vi "CRYDataView Pic LIB.vi"(7 "sAction":string, 8 "nData":i32, 9 "sData":string, 10 "sOption":string, 11 "cView":T1) -> (0 "nData_Out":i32, 1 "sData_Out":string, 3 "cView_Out":T1)   [LabVIEW 2013]
uses:
  Control/CRYGraph Property.ctl
  SubVI/CRYMain Sub Window Global.vi
  CRYMainGlobal.vi
  CRYProject/CRYProject Editor Global.vi
panel:
  in  "bWait":bool=TRUE
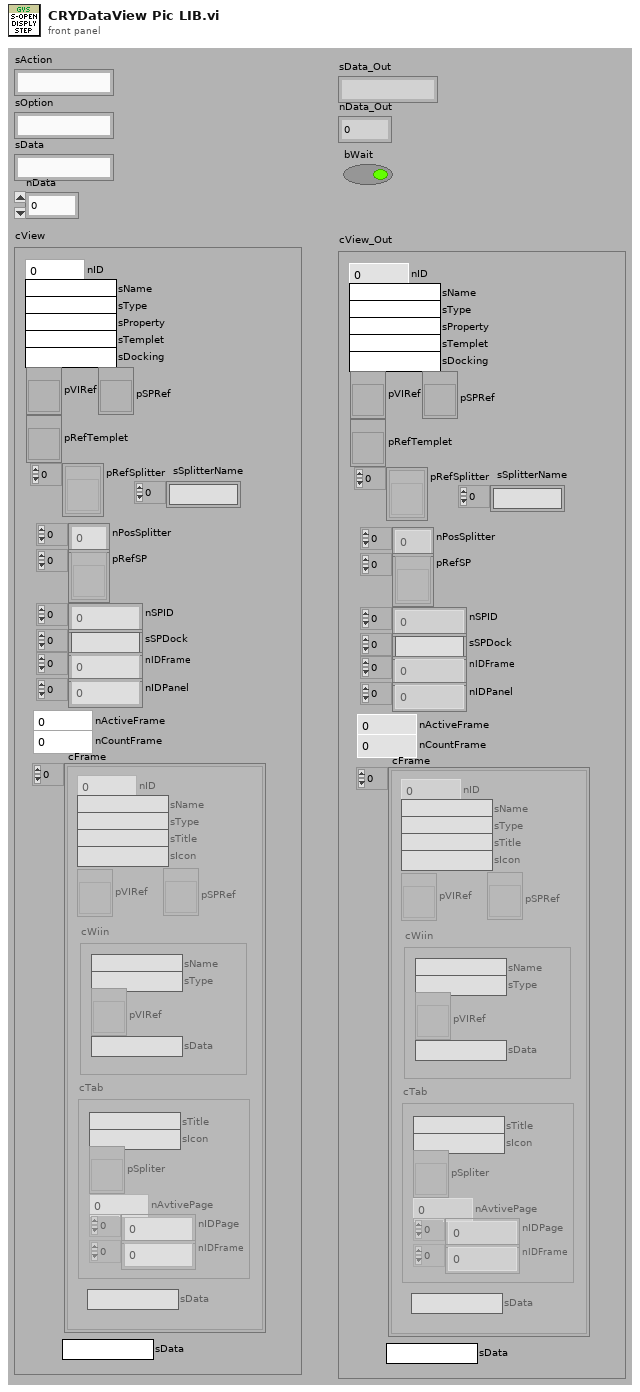
[diagram p1: front panel]
types:
  T1 = cluster{"nID":i32, "sName":string, "sType":string, "sProperty":string, "sTemplet":string, "sDocking":string, "pVIRef":refnum<vi>, "pSPRef":refnum<vi>, "pRefTemplet":refnum<vi>, "pRefSplitter":refnum<vi>[], "nPosSplitter":i32[], "pRefSP":refnum<vi>[], "nSPID":i32[], "sSPDock":string[], "nIDFrame":i32[], "nIDPanel":i32[], "nActiveFrame":i32, "nCountFrame":i32, "cFrame":cluster{"nID":i32, "sName":string, "sType":string, "sTitle":string, "sIcon":string, "pVIRef":refnum<vi>, "pSPRef":refnum<vi>, "cWiin":cluster{"sName":string, "sType":string, "pVIRef":refnum<vi>, "sData":string}, "cTab":cluster{"sTitle":string, "sIcon":string, "pSpliter":refnum<vi>, "nAvtivePage":i32, "nIDPage":i32[], "nIDFrame":i32[]}, "sData":string}[], "sData":string, "sSplitterName":string[]}
  T2 = typedef "CRYGraph Property.ctl" = cluster{"LegendShow":bool, "Legend Splitter Position":dbl, "Data Names":string[], "Item Symbols":i32[], "Color Array":u32[], "Flattened Plot Property":string, "CursorShow":bool, "Flattened Cursor Property":string, "Graph Number":i32, "Flattened Scale Property":string, "PreviewShow":bool, "MagnitudeShow":bool, "PaletteShow":bool, "XYShow":bool, "FrequencyShow":bool, "Frequency Splitter Position":dbl, "XYGraph Splitter Position":dbl, "Frequency Symbols":i32[], "LegendVScrollShow":bool, "FrequencyVScrollShow":bool, "PhaseShow":bool, "Title Name":string}
  T3 = typedef "LVRectTypeDef.ctl" = cluster{"Left":i16, "Top":i16, "Right":i16, "Bottom":i16}
  T4 = cluster{"nID":i32[], "Frame":cluster{"nType":i32, "nParent":i32, "pVIW":refnum<vi>, "pSPW":refnum<vi>, "nTypeF":i32, "pVIF":refnum<vi>, "pSPF":refnum<vi>, "nIDSpliter":i32, "nProperty":i32, "Bound":T3, "nID":i32, "nData":i32, "sData":string, "pWVI":refnum<vi>, "sTitle":string, "cPages":cluster{"nPage":i32, "sTitle":string, "sIcon":string, "pVI":refnum<vi>, "nID":i32}[], "pTab":refnum<vi>, "nIDPages":i32[], "pSPT":refnum<vi>, "sTemp":string, "nDockID":i32, "nDockLR":i32, "sIcon":string}[]}
  T5 = cluster{"nType":i32, "nParent":i32, "pVIW":refnum<vi>, "pSPW":refnum<vi>, "nTypeF":i32, "pVIF":refnum<vi>, "pSPF":refnum<vi>, "nIDSpliter":i32, "nProperty":i32, "Bound":T3, "nID":i32, "nData":i32, "sData":string, "pWVI":refnum<vi>, "sTitle":string, "cPages":cluster{"nPage":i32, "sTitle":string, "sIcon":string, "pVI":refnum<vi>, "nID":i32}[], "pTab":refnum<vi>, "nIDPages":i32[], "pSPT":refnum<vi>, "sTemp":string, "nDockID":i32, "nDockLR":i32, "sIcon":string}[]
  T6 = typedef "CRYTS.ctl" = cluster{"No.TS":u16, "TS File Path":path, "TS Name":string, "EditStepName":string, "Steps":T7[], "New State":bool, "Change State":bool, "Flattened CurveLib Data":string, "Document Data":string, "EditStepNo":u16, "Operator Start File":string, "Sequence Type":string, "Sequence Language":string}
  T7 = typedef "CRYStep.ctl" = cluster{"No.VI":i32, "Category":string, "StepName":string, "Seq setup flattened":string, "Comment":string, "Steps config.":bool[], "Jump config":i32[], "Start":dbl, "Increment":dbl, "Name":string, "Unit":string, "Y data":u16, "Y prefix":string, "Y dB ref":dbl, "Y unit":string, "Repeat State Array":cluster{"Start":dbl, "Increment":dbl, "Count":i32, "Num":i32}[]}
  T8 = cluster{"nType":i32, "nParent":i32, "pVIW":refnum<vi>, "pSPW":refnum<vi>, "nTypeF":i32, "pVIF":refnum<vi>, "pSPF":refnum<vi>, "nIDSpliter":i32, "nProperty":i32, "Bound":T3, "nID":i32, "nData":i32, "sData":string, "pWVI":refnum<vi>, "sTitle":string, "cPages":cluster{"nPage":i32, "sTitle":string, "sIcon":string, "pVI":refnum<vi>, "nID":i32}[], "pTab":refnum<vi>, "nIDPages":i32[], "pSPT":refnum<vi>, "sTemp":string, "nDockID":i32, "nDockLR":i32, "sIcon":string}
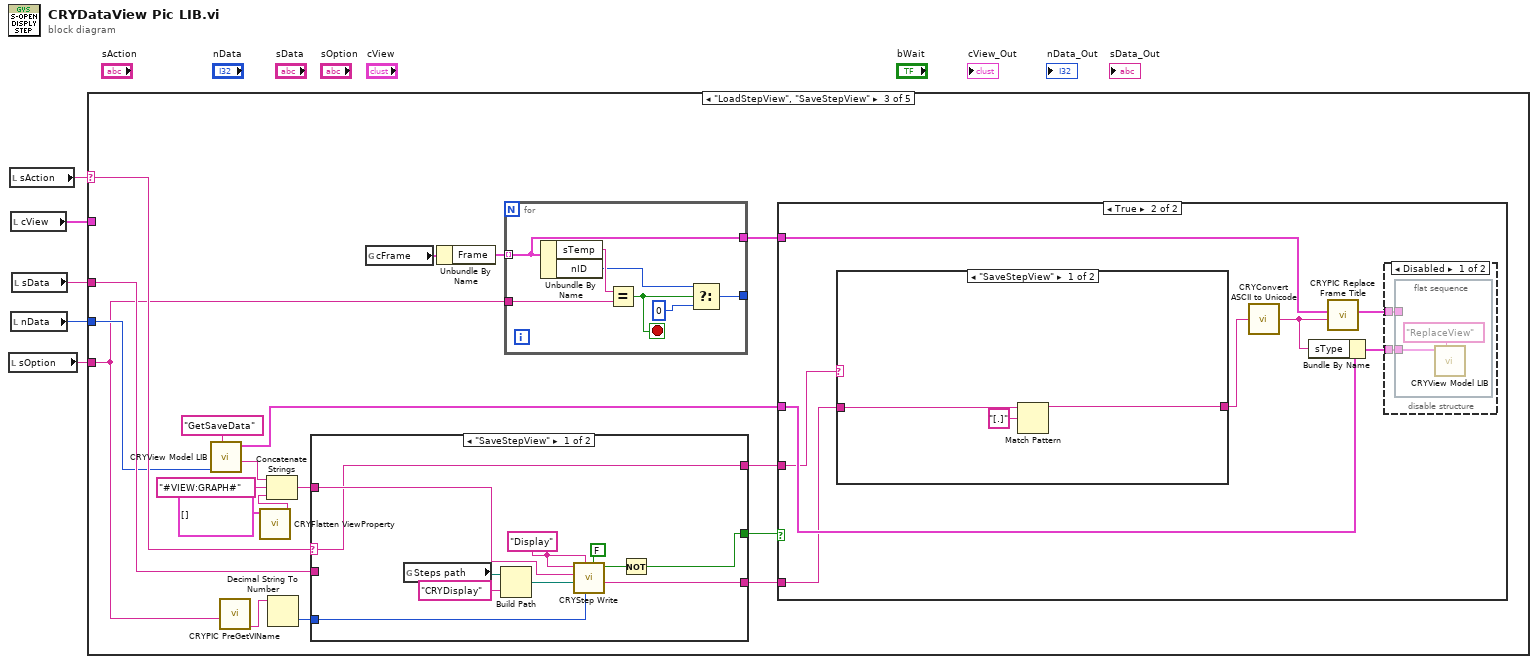
[diagram p0: block diagram]
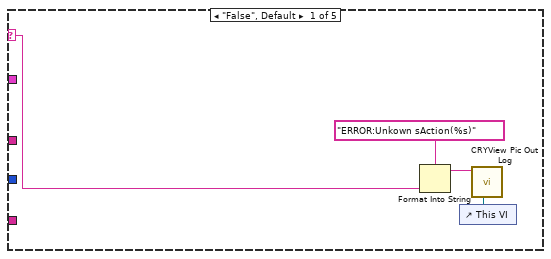
[diagram p2: hidden frame]
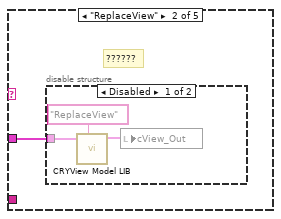
[diagram p3: hidden frame]
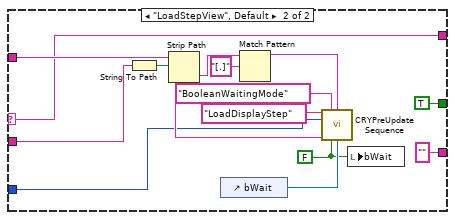
[diagram p5: hidden frame]
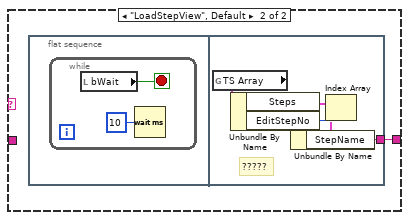
[diagram p8: hidden frame]
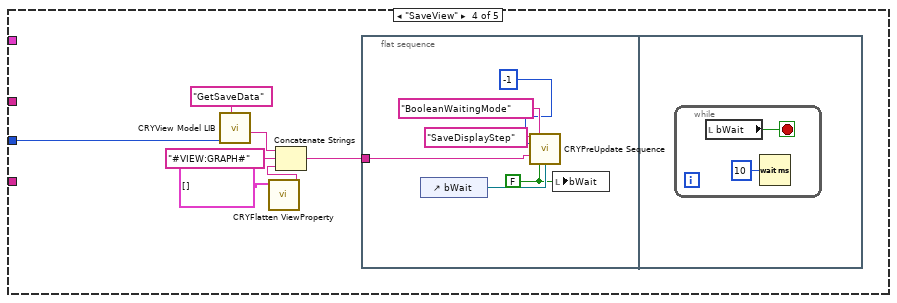
[diagram p9: hidden frame]
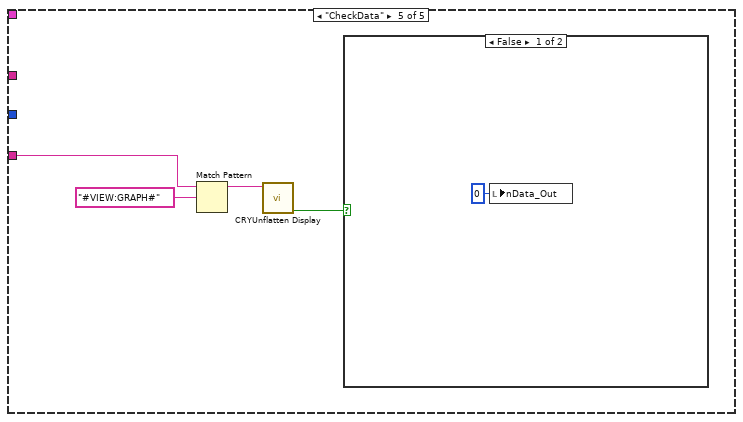
[diagram p10: hidden frame]
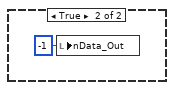
[diagram p11: hidden frame]
diagram:
  n1 = local read "sOption"() -> (w2:string)
  n2 = local read "sAction"() -> (w5:string)
  n3 = local read "cView"() -> (w1:T1)
  n4 = local read "nData"() -> (w3:i32)
  n5 = local read "sData"() -> (w4:string)
  n6 = case shown="\"LoadStepView\", \"SaveStepView\"" w5 {
    selector: w5 -> [w7 _ w28 _ _]
    tunnel: w4 -> [_ _ w29 _ _]
    tunnel: w3 -> [_ _ w22 w89 _]
    tunnel: w2 -> [_ _ w17 _ w105]
    tunnel: w1 -> [_ w10 _ _ _]
    frame "False", Default {
      n7 = Format Into String(format string="ERROR:Unkown sAction(%s)", w7) -> (resulting string=w6:string)  [unwired: 2 in, 1 out]
      n8 = control-ref of="This VI"() -> (w9:refnum<vi>)
      n9 = call "CRYView Pic Out Log.vi"("vi reference"=w9, "sData"=w6) -> ()  [unwired: 10 in]
    }
    frame "ReplaceView" {
      # "??????"
      n10 = disable-structure shown="Disabled" {
        disable-tunnel: w10 -> [w13 _]
        frame Disabled {
          n11 = call "CRYView Model LIB.vi"("sAction"="ReplaceView", "cView"=w13) -> ("cView_Out"=w11:T1)  [unwired: 7 in, 2 out]
          n12 = local write "cView_Out"(w11) -> ()
        }
        frame Enabled {
        }
      }
    }
    frame "LoadStepView", "SaveStepView" {
      n13 = call "CRYView Model LIB.vi"("sAction"="GetSaveData", "nData"=w22) -> ("sData_Out"=w27:string, "cView_Out"=w19:T1)  [unwired: 7 in, 1 out]
      n14 = call "CRYPIC PreGetVIName.vi"("sVIName"=w17) -> ("sData_Out"=w16:string)  [unwired: 9 in, 1 out]
      n15 = call "CRYFlatten ViewProperty.vi"("GraphViewProperty"=T2[] []) -> ("ViewPro flattened"=w25:string)  [unwired: 10 in]
      n16 = Concatenate Strings(w27, "#VIEW:GRAPH#" ("regular expression"), w25) -> (w21:string)
      n17 = Decimal String To Number(string=w16) -> (number=w18:i32)  [unwired: 2 in, 1 out]
      n18 = case shown="\"SaveStepView\"" w28 {
        selector: w28 -> [w33 w44]
        tunnel: [w36 TRUE] -> w20
        tunnel: w21 -> [w39 w52]
        tunnel: w29 -> [_ w50]
        tunnel: w18 -> [w38 w46]
        tunnel: [w35 "" ("name")] -> w15
        tunnel: [w33 w44] -> w14
        frame "SaveStepView" {
          w40 = "Display" ("Step File Name")
          n19 = global read "CRYMainGlobal.vi" "Steps path"() -> (w42:path)
          n20 = Build Path(base path=w42, name or relative path="CRYDisplay") -> (appended path=w41:path)
          n21 = call "CRYStep Write.vi"("Default"=FALSE, "Proper VI No"=w38, "Category Name"=w40, "Step File Path"=w41, "Step flattened"=w39, "Step File Name"=w40) -> ("name"=w35:string, "Cancel"=w37:bool)  [unwired: 3 in, 1 out]
          n22 = Not(x=w37) -> (.not. x?=w36:bool)
        }
        frame "LoadStepView", Default {
          w56 = FALSE ("AllChangeFlg")
          n23 = String To Path(string=w50) -> (path=w51:path)
          n24 = Strip Path(path=w51) -> (name=w48:string)  [unwired: 1 out]
          n25 = control-ref of="bWait"() -> (w57:refnum<vi>)
          n26 = Match Pattern(string=w48, regular expression="[.]") -> (before substring=w47:string)  [unwired: 4 out]
          n27 = call "CRYPreUpdate Sequence.vi"("EventName"="LoadDisplayStep", "Mode"="BooleanWaitingMode", "StepName Arg3"=w47, "Proper VI No"=w46, "Step flattened Arg2"=w52, "AllChangeFlg"=w56, "Ref Variant"=w57) -> ()  [unwired: 9 in]
          n28 = local write "bWait"(w56) -> ()
        }
      }
      n29 = global read "CRYMain Sub Window Global.vi" "cFrame"() -> (w31:T4)
      n30 = Unbundle By Name(w31) -> ("Frame"=w30:T5)
      n31 = for {
        tunnel: w30 -> [w85] mode=indexing
        tunnel: w17 -> [w86]
        tunnel: [w85] -> w32
        tunnel: [w81] -> _
        stop <- w84 stop-if-true
        n32 = Unbundle By Name(w85) -> ("sTemp"=w87:string, "nID"=w83:i32)
        n33 = Equal?(x=w87, y=w86) -> (x = y?=w84:bool)
        n34 = Select(t=w83, s=w84, f=0) -> (s? t:f=w81:i32)
      }
      n35 = case shown="True" w20 {
        tunnel: w32 -> [_ w65]
        tunnel: w19 -> [_ w62]
        tunnel: w15 -> [_ w59]
        tunnel: w14 -> [_ w58]
        frame False {
        }
        frame True {
          n36 = case shown="\"SaveStepView\"" w58 {
            tunnel: [w70 w73] -> w60
            tunnel: w59 -> [w71 _]
            frame "SaveStepView" {
              n37 = Match Pattern(string=w71, regular expression="[.]") -> (before substring=w70:string)  [unwired: 4 out]
            }
            frame "LoadStepView", Default {
              n38 = flat-sequence {
                tunnel: [w76] -> w73
                frame #0 {
                  n39 = while {
                    stop <- w75 stop-if-true
                    n40 = local read "bWait"() -> (w75:bool)
                    n41 = Wait (ms)(milliseconds to wait=u32 10) -> ()  [unwired: 1 out]
                  }
                }
                frame #1 {
                  # "?????"
                  n42 = global read "CRYProject Editor Global.vi" "TS Array"() -> (w77:T6)
                  n43 = Unbundle By Name(w77) -> ("Steps"=w78:T7[], "EditStepNo"=w80:u16)
                  n44 = Index Array(array=w78, index=w80) -> (element=w79:T7)
                  n45 = Unbundle By Name(w79) -> ("StepName"=w76:string)
                }
              }
            }
          }
          n46 = call "CRYConvert ASCII to Unicode.vi"("ASCII"=w60) -> ("Unicode"=w63:string)  [unwired: 4 in]
          n47 = Bundle By Name(cluster=w62, "sType"=w63) -> (w61:T1)
          n48 = call "CRYPIC Replace Frame Title.vi"("sNewTitle"=w63, "tFrame"=w65) -> ("tFrame_Out"=w64:T8)  [unwired: 9 in]
          n49 = disable-structure shown="Disabled" {
            disable-tunnel: w64 -> [w67 _]
            disable-tunnel: w61 -> [w66 _]
            frame Disabled {
              n50 = flat-sequence {
                tunnel: w67 -> [_]
                tunnel: w66 -> [w68]
                frame #0 {
                  n51 = call "CRYView Model LIB.vi"("sAction"="ReplaceView", "cView"=w68) -> ()  [unwired: 7 in, 3 out]
                }
              }
            }
            frame Enabled {
            }
          }
        }
      }
    }
    frame "SaveView" {
      n52 = call "CRYView Model LIB.vi"("sAction"="GetSaveData", "nData"=w89) -> ("sData_Out"=w94:string)  [unwired: 7 in, 2 out]
      n53 = call "CRYFlatten ViewProperty.vi"("GraphViewProperty"=T2[] []) -> ("ViewPro flattened"=w92:string)  [unwired: 10 in]
      n54 = Concatenate Strings(w94, "#VIEW:GRAPH#" ("regular expression"), w92) -> (w88:string)
      n55 = flat-sequence {
        tunnel: w88 -> [w100]
        frame #0 {
          w98 = FALSE ("AllChangeFlg")
          n56 = control-ref of="bWait"() -> (w99:refnum<vi>)
          n57 = call "CRYPreUpdate Sequence.vi"("EventName"="SaveDisplayStep", "Mode"="BooleanWaitingMode", "Proper VI No"=-1, "Project View Step Name Identifier Arg1"=w100, "AllChangeFlg"=w98, "Ref Variant"=w99) -> ()  [unwired: 10 in]
          n58 = local write "bWait"(w98) -> ()
        }
        frame #1 {
          n59 = while {
            stop <- w102 stop-if-true
            n60 = local read "bWait"() -> (w102:bool)
            n61 = Wait (ms)(milliseconds to wait=u32 10) -> ()  [unwired: 1 out]
          }
        }
      }
    }
    frame "CheckData" {
      n62 = Match Pattern(string=w105, regular expression="#VIEW:GRAPH#") -> (before substring=w104:string)  [unwired: 1 in, 3 out]
      n63 = call "CRYUnflatten Display.vi"("Flatten Display"=w104) -> ("Error?"=w103:bool)  [unwired: 8 in, 2 out]
      n64 = case shown="False" w103 {
        frame False {
          n65 = local write "nData_Out"(0 ("nData_Out")) -> ()
        }
        frame True {
          n66 = local write "nData_Out"(-1 ("nData_Out")) -> ()
        }
      }
    }
  }
